vi "1motorPwm (SubVI).vi"(7 "Motor ID":T1, 8 "error in (no error)":errorcluster, 10 "motorPwmSpeed":dbl, 11 "TitanQuad in":refnum<class "TitanQuad.lvclass">) -> (0 "error out":errorcluster, 3 "TitanQuad out":refnum<class "TitanQuad.lvclass">)   [LabVIEW 2020]
uses:
  <vilib>/CISH Robotics/L4VMX TitanQuad/TitanQuad.lvclass
  <vilib>/CISH Robotics/L4VMX TitanQuad/Motor ID.ctl
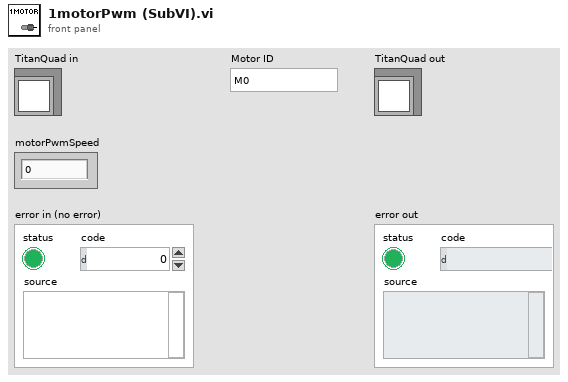
[diagram p1: front panel]
types:
  T1 = typedef "TitanQuad.lvlib/TitanQuad.lvclass/Motor ID.ctl" = enum16{"M0", "M1", "M2", "M3"}
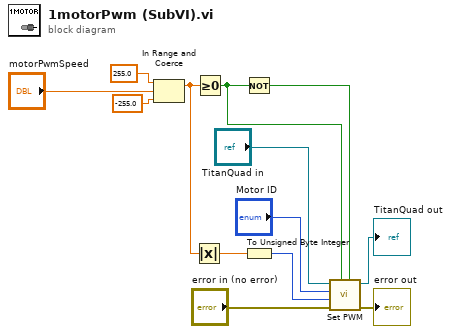
[diagram p0: block diagram]
diagram:
  n1 = In Range and Coerce(upper limit=255.0, x="motorPwmSpeed", lower limit=-255.0) -> (coerced(x)=w10:dbl)  [unwired: 1 out]
  n2 = Absolute Value(x=w10) -> (abs(x)=w6:dbl)
  n3 = Greater Or Equal To 0?(x=w10) -> (x >= 0?=w4:bool)
  n4 = Not(x=w4) -> (.not. x?=w5:bool)
  n5 = To Unsigned Byte Integer(number=w6) -> (unsigned 8bit integer=w7:u8)
  n6 = call <vilib>:"Set PWM.vi"("Dir B"=w5, "Dir A"=w4, "Error In"="error in (no error)", "Duty Cycle (0~255)"=w7, "Motor ID"="Motor ID", "TitanQuad Object"="TitanQuad in") -> ("Error Out"=→"error out":errorcluster, "TitanQuad Object"=→"TitanQuad out":refnum<class "TitanQuad.lvclass">)  [unwired: 4 in]
